vi "test1-SystemLevelModuleInListModuleAPI.vi"(8 "error in (no error)":errorcluster, 11 "TestCase in":refnum<class "testcase-CSMSystemLevelModule.lvclass">) -> (0 "error out":errorcluster, 3 "TestCase out":refnum<class "testcase-CSMSystemLevelModule.lvclass">)   [LabVIEW 2017, in "testcase-CSMSystemLevelModule.lvclass"]
uses:
  testcase-CSMSystemLevelModule.lvclass
  src/user.lib/_NEVSTOP/Communicable State Machine(CSM)/_Support/Typedef/_CSM_List Module Scope.ctl
  <vilib>/addons/_JKI Toolkits/VI Tester/TestCase.llb/TestCase.lvclass
  src/user.lib/_NEVSTOP/Communicable State Machine(CSM)/Communicable State Machine.lvlib
  C:/Program Files (x86)/National Instruments/LabVIEW 2017/vi.lib/addons/_JKI Toolkits/VI Tester/TestCase.llb/TestCase.lvclass
panel:
  out "error out 2":errorcluster
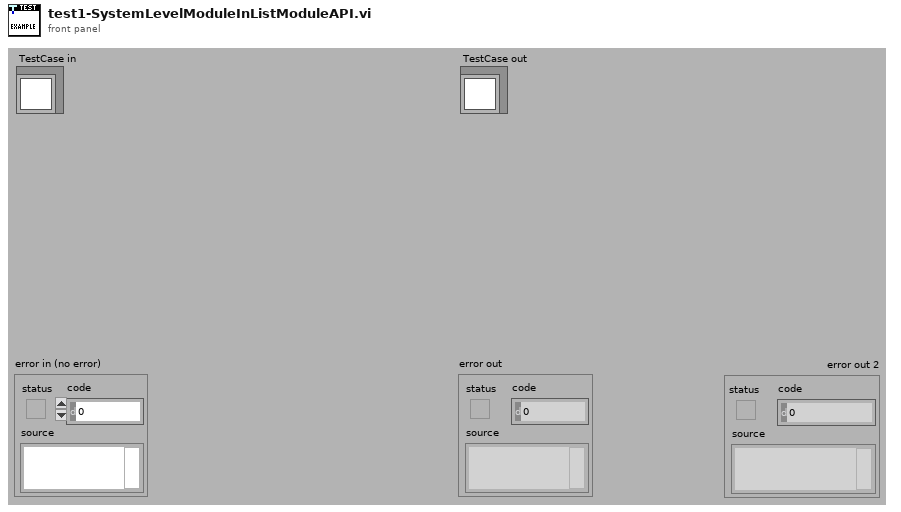
[diagram p1: front panel]
types:
  T1 = typedef "Communicable State Machine.lvlib/_CSM_List Module Scope.ctl" = enum16{"Normal", "System Only", "All"}
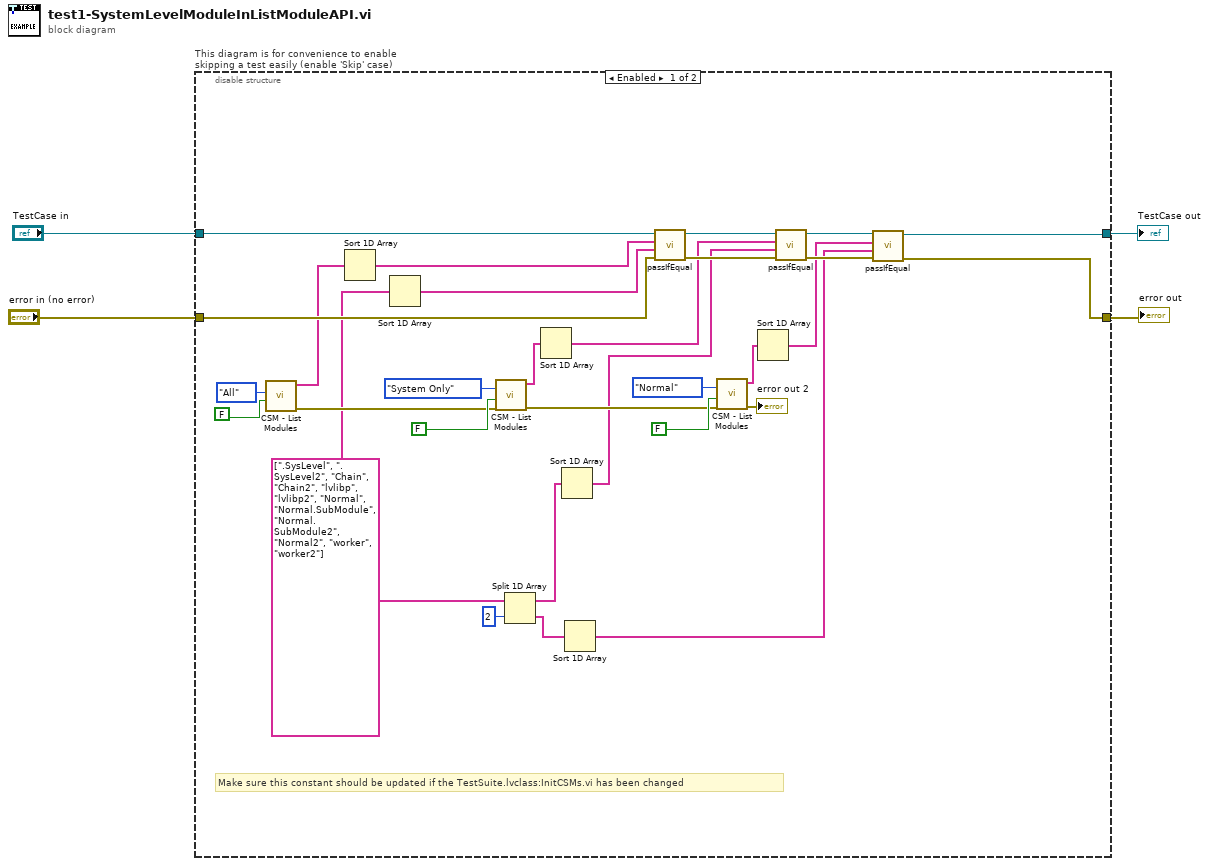
[diagram p0: block diagram]
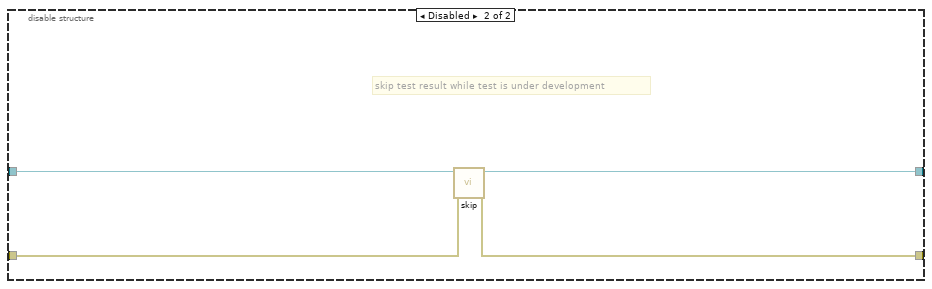
[diagram p2: hidden frame]
diagram:
  n1 = disable-structure "This diagram is for convenience to enable skipping a test easily (enable 'Skip' case)" shown="Enabled" {
    disable-tunnel: "TestCase in" -> [w28 w38]
    disable-tunnel: [w19 w36] -> w1
    disable-tunnel: [w16 w37] -> w3
    disable-tunnel: "error in (no error)" -> [w27 w35]
    frame Enabled {
      w12 = string[] [".SysLevel", ".SysLevel2", "Chain", "Chain2", "lvlibp", "lvlibp2", "Normal", "Normal.SubModule", "Normal.SubModule2", "Normal2", "worker", "worker2"] ("Module Names in All Scope")
      # "Make sure this constant should be updated if the TestSuite.lvclass:InitCSMs.vi has been changed"
      n2 = call "CSM - List Modules.vi"("With Nodes? (F)"=FALSE, "Scope (Normal)"=_CSM_List_Module_Scope."All") -> ("error out"=w26:errorcluster, "Module Names"=w24:string[])  [unwired: 8 in]
      n3 = Sort 1D Array(array=w24) -> (sorted array=w23:string[])
      n4 = Sort 1D Array(array=w12) -> (sorted array=w22:string[])
      n5 = call "CSM - List Modules.vi"("Error In"=w26, "With Nodes? (F)"=FALSE, "Scope (Normal)"=_CSM_List_Module_Scope."System Only") -> ("error out"=w25:errorcluster, "Module Names"=w15:string[])  [unwired: 7 in]
      n6 = Split 1D Array(array=w12, index=2) -> (first subarray=w10:string[], second subarray=w9:string[])
      n7 = Sort 1D Array(array=w15) -> (sorted array=w14:string[])
      n8 = Sort 1D Array(array=w10) -> (sorted array=w13:string[])
      n9 = Sort 1D Array(array=w9) -> (sorted array=w6:string[])
      n10 = call-dynamic "passIfEqual.vi"("error in (no error)"=w27, "y"=w22, "x"=w23, "TestCase in"=w28) -> ("error out"=w18:errorcluster, "TestCase out"=w21:refnum<class "testcase-CSMSystemLevelModule.lvclass">)  [unwired: 6 in]
      n11 = call "CSM - List Modules.vi"("Error In"=w25, "With Nodes? (F)"=FALSE, "Scope (Normal)"=_CSM_List_Module_Scope."Normal") -> ("error out"=→"error out 2":errorcluster, "Module Names"=w8:string[])  [unwired: 7 in]
      n12 = Sort 1D Array(array=w8) -> (sorted array=w7:string[])
      n13 = call-dynamic "passIfEqual.vi"("error in (no error)"=w18, "y"=w13, "x"=w14, "TestCase in"=w21) -> ("error out"=w17:errorcluster, "TestCase out"=w20:refnum<class "testcase-CSMSystemLevelModule.lvclass">)  [unwired: 6 in]
      n14 = call-dynamic "passIfEqual.vi"("error in (no error)"=w17, "y"=w6, "x"=w7, "TestCase in"=w20) -> ("error out"=w16:errorcluster, "TestCase out"=w19:refnum<class "testcase-CSMSystemLevelModule.lvclass">)  [unwired: 6 in]
    }
    frame Disabled {
      # "skip test result while test is under development"
      n15 = call <vilib>:"skip.vi"("error in (no error)"=w35, "TestCase in"=w38) -> ("error out"=w37:errorcluster, "TestCase out"=w36:refnum<class "testcase-CSMSystemLevelModule.lvclass">)  [unwired: 8 in]
    }
  }
  "error out" <- w3
  "TestCase out" <- w1
